vi "Extract F0.vi"(8 "Error In":errorcluster) -> (0 "Error Out":errorcluster)   [LabVIEW 2018, in "AnalysisSupport.lvlib"]
uses:
  AnalysisSupport.lvlib
  Analysis Support/Controls/F0 Extraction Test Types.ctl
  Analysis Support/Controls/F0 Extraction States.ctl
  Analysis Support/Controls/F0 Cluster.ctl
  <vilib>/Waveform/WDTOps.llb/WDT Get Waveform Subset DBL.vi
  <vilib>/Analysis/NI_AALBase.lvlib
  CollectionSupport.lvlib
panel:
  out "Selected":dbl format="%#.2g"
  out "Test-Matched Files":path[](array[path])
  out "Min":dbl
  out "Max":dbl
  out "Median":dbl
  out "Progress Bar":u8(slide) scale=0.0..10.0
  out "F0 Array (Hz)":dbl[](array[numeric]) format="%#.2g"
  out "CoV":dbl format="%.2f%%"
  out "St.Dev":dbl format="%#.2g"
  out "Mean F0 (Hz)":dbl format="%#.2g"
  in  "Trial":dbl=1.0 min=1.0 max=15.0 step=1.0
  in  "Section Duration":dbl=0.1 min=0.1 max=1.0 step=0.1
  in  "Start Second":dbl min=0.0 max=10.0 step=0.1
  in  "Remove Button":bool
  in  "ReRun Button":bool
  in  "Save  Button":bool
  in  "Test Type Select":T1 items=["Labial SGP", "Labial PTP", "Mech Mouth", "Mech Mask"]
  in  "Trial Number":i32=1 min=1 max=15 step=1
  in  "Exit Button":bool
  in  "Open Button":bool
  in  "Examine Button":bool
  in  "Extract Button":bool
  out "Audio Graph":dynamicdata(graph)
  out "Total Files":i32
  out "All Files in Directory":path[](array[path])
  # "Remove an index to change stats"
  # "Save the mean, standard deviation, & coefficient of variation to a txt file."
  # "Re-run extraction using a different section of signal"
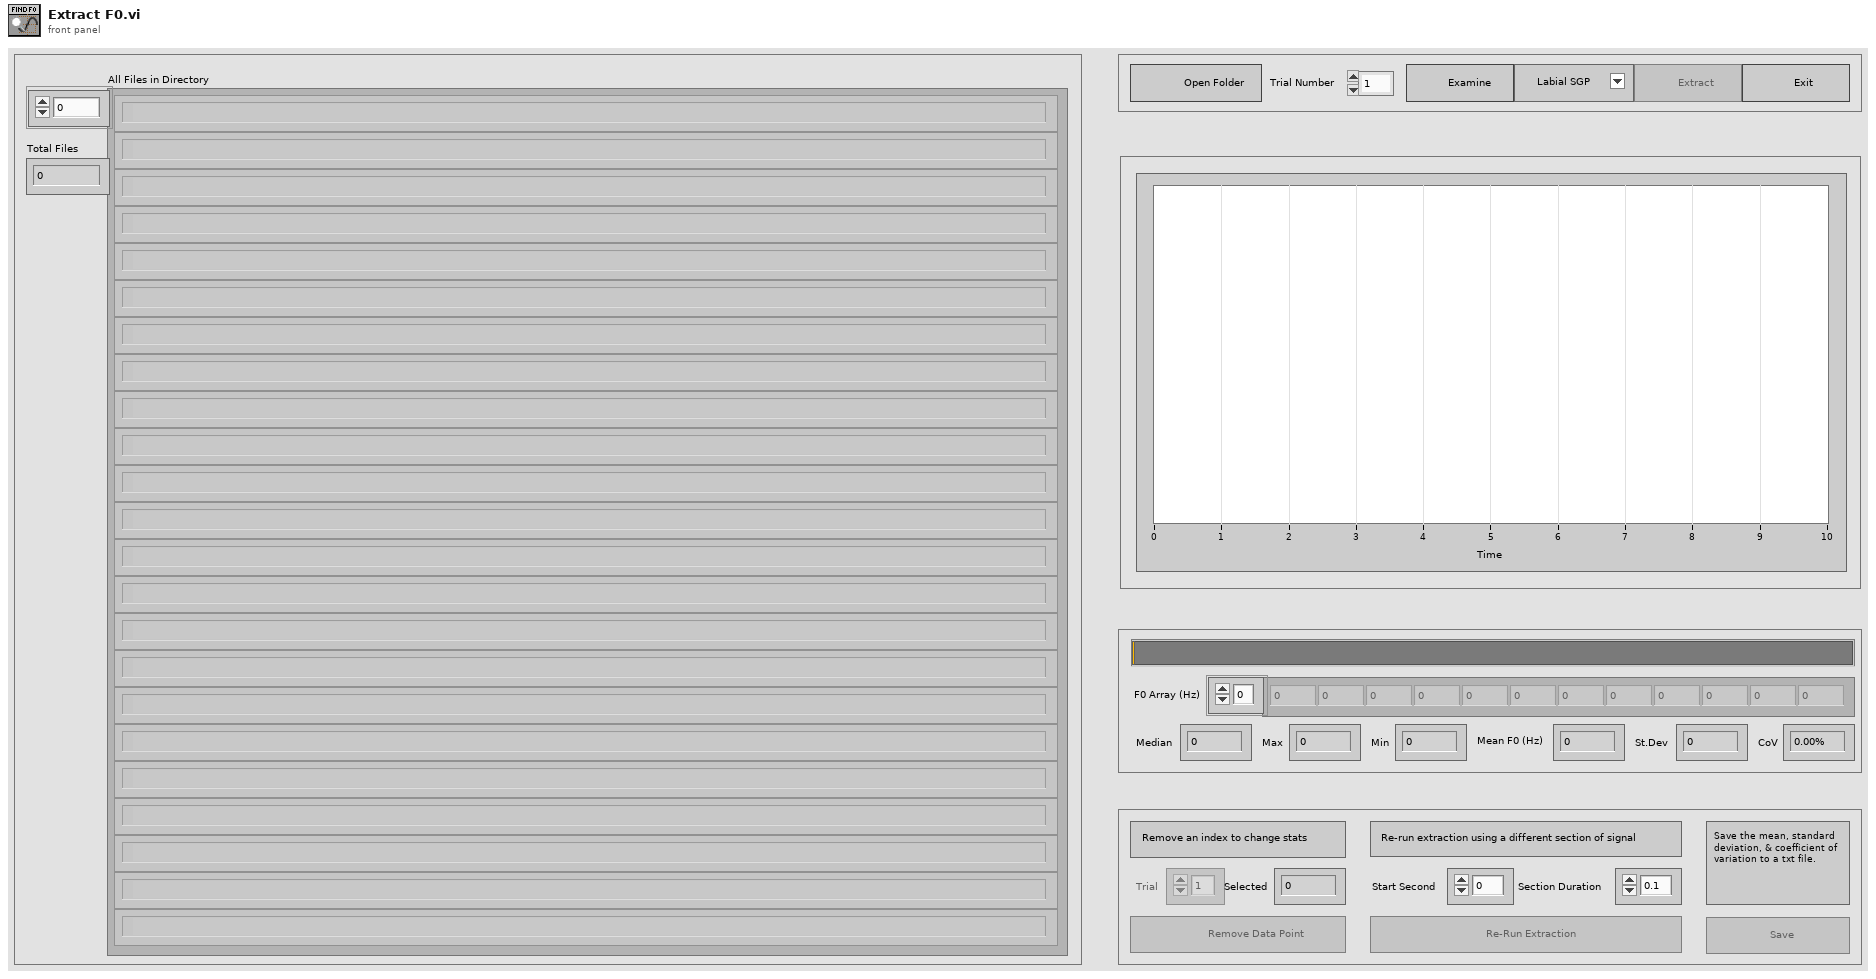
[diagram p1: front panel]
types:
  T1 = typedef "AnalysisSupport.lvlib/F0 Extraction Test Types.ctl" = u16
  T2 = typedef "AnalysisSupport.lvlib/F0 Cluster.ctl" = cluster{"F0 and Trial #":cluster{"F0 Array":dbl[], "Matched Trial #":string[]}, "Mean":dbl, "STD":dbl, "CoV":dbl, "Median":dbl, "Max":dbl, "Min":dbl, "Start Second":dbl, "Section Duration":dbl, "Total Files":i32, "Trial Number":i32, "Progress Bar Max":u8, "Selected F0":dbl, "Trial Index":dbl, "Test Type":string, "File Array":path[], "File Subset":path[], "Audio Data":dynamicdata, "References":cluster{"Trial":refnum<vi>, "Open Button":refnum<vi>, "Examine Button":refnum<vi>, "Test Type Select":refnum<vi>, "Extract Button":refnum<vi>, "Exit Button":refnum<vi>, "Remove Button":refnum<vi>, "ReRun Button":refnum<vi>, "Save  Button":refnum<vi>, "Progress Bar":refnum<vi>}}
  T3 = typedef "AnalysisSupport.lvlib/F0 Extraction States.ctl" = enum16{"Initialize", "Update", "Wait", "Open Folder", "Examine", "Extract", "Re Run", "Remove", "Save", "Exit"}
  T4 = enum8{"Enabled", "Disabled", "Disabled and Grayed Out"}
  T5 = enum16{"open", "replace", "create", "open or create", "replace or create", "replace or create with confirmation"}
  T6 = cluster{"Trial":refnum<vi>, "Open Button":refnum<vi>, "Examine Button":refnum<vi>, "Test Type Select":refnum<vi>, "Extract Button":refnum<vi>, "Exit Button":refnum<vi>, "Remove Button":refnum<vi>, "ReRun Button":refnum<vi>, "Save  Button":refnum<vi>, "Progress Bar":refnum<vi>}
  T7 = cluster{"F0 Array":dbl[], "Matched Trial #":string[]}
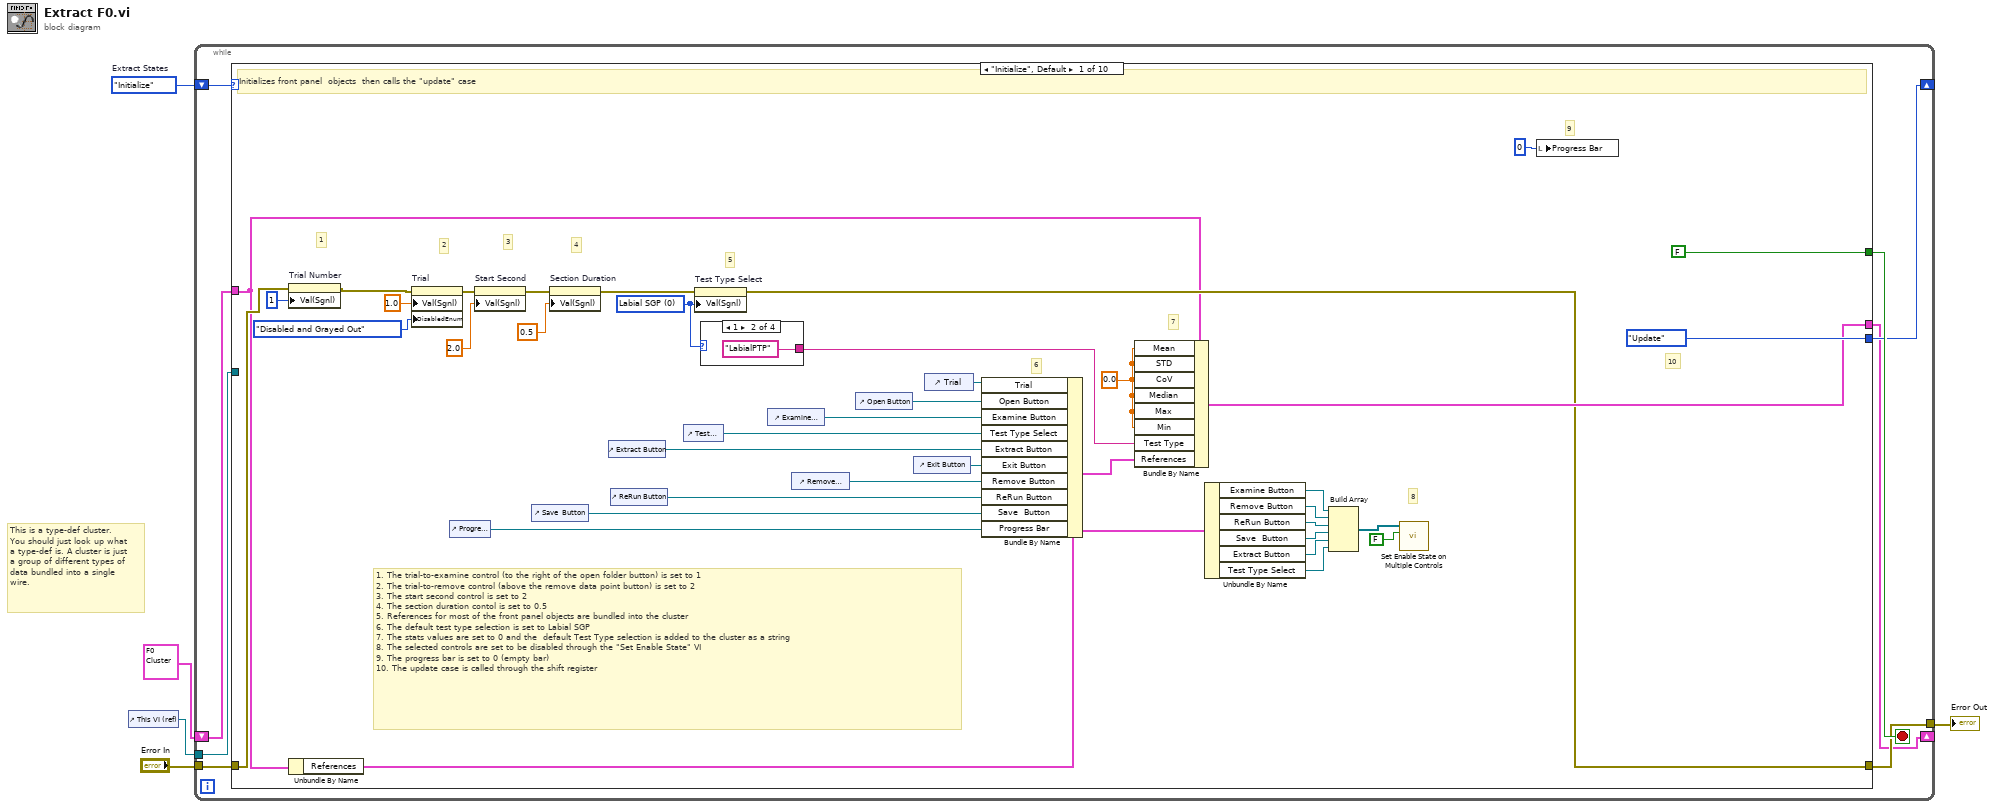
[diagram p0: block diagram]
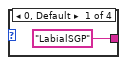
[diagram p2: hidden frame]
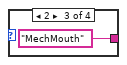
[diagram p3: hidden frame]
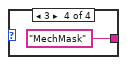
[diagram p4: hidden frame]
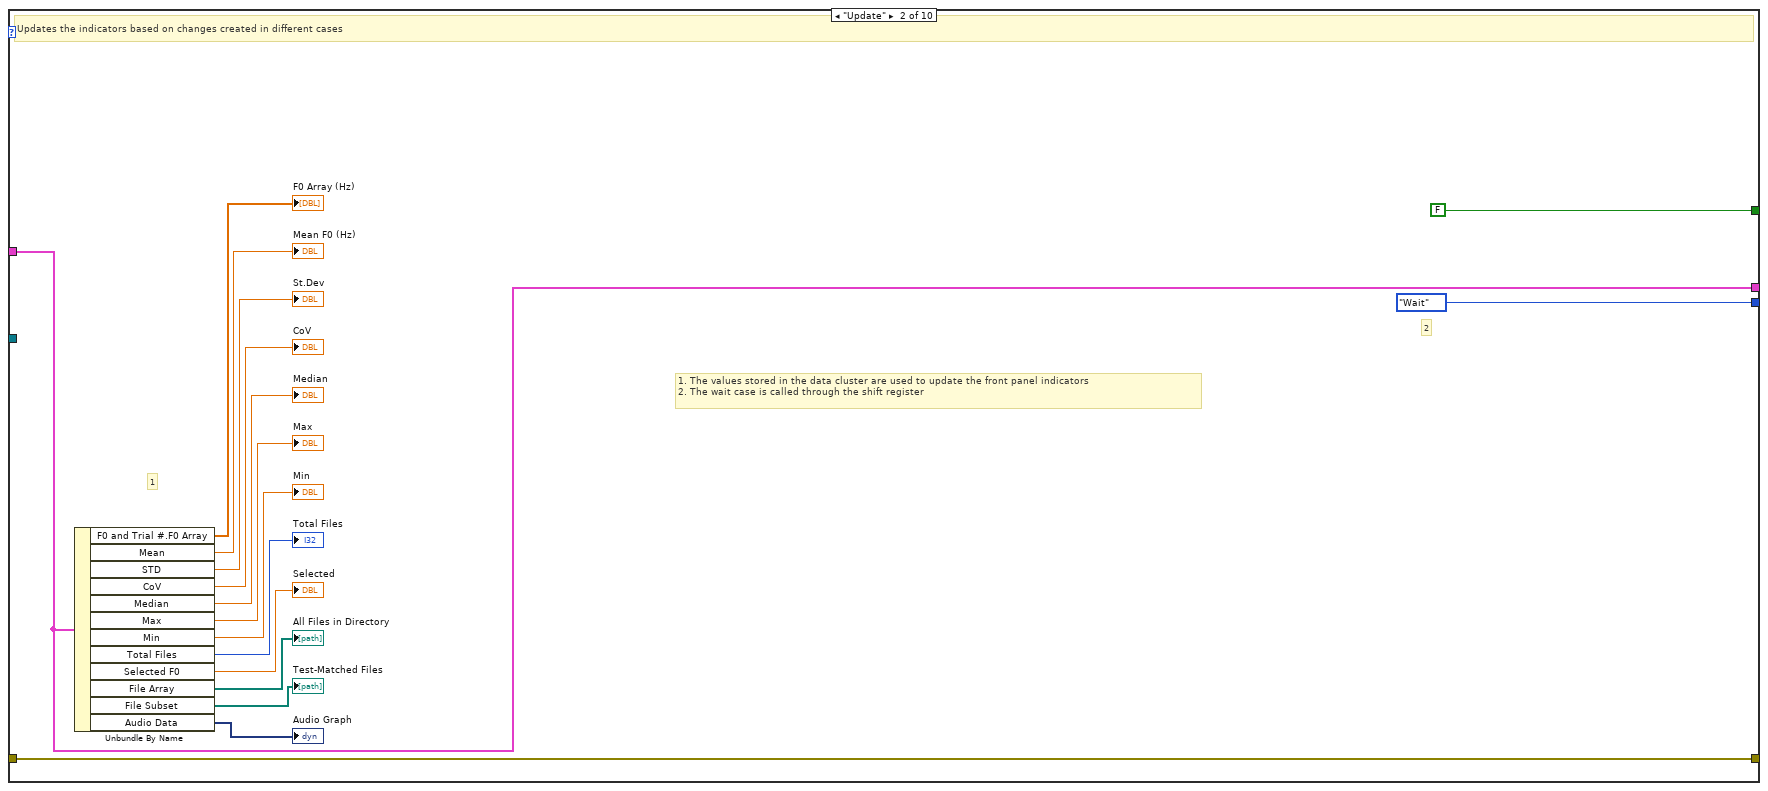
[diagram p5: hidden frame]
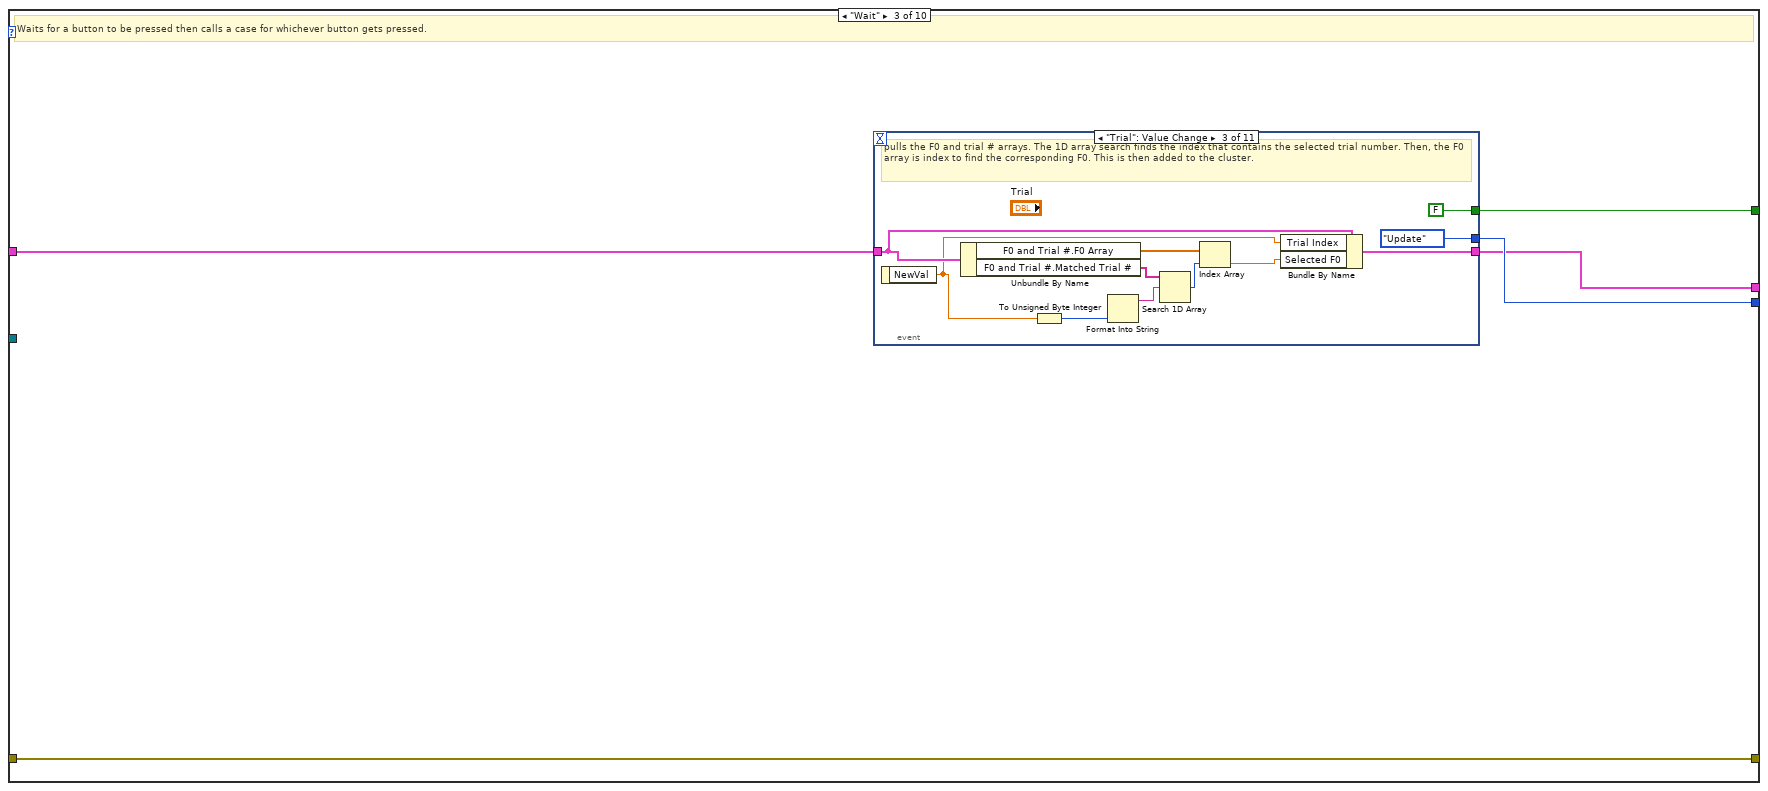
[diagram p6: hidden frame]
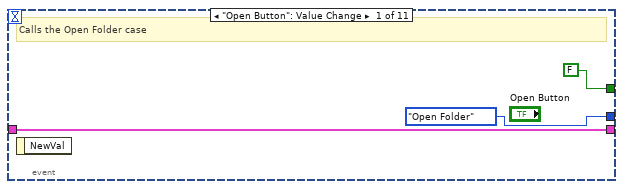
[diagram p7: hidden frame]
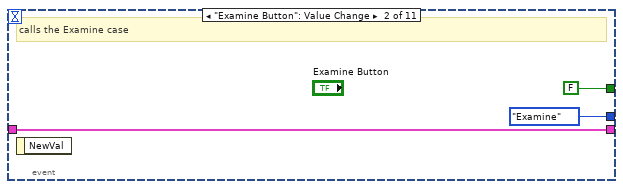
[diagram p8: hidden frame]
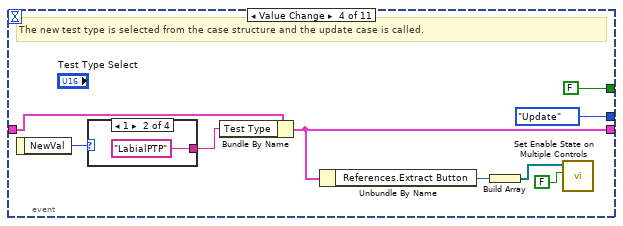
[diagram p9: hidden frame]
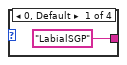
[diagram p10: hidden frame]
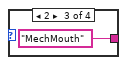
[diagram p11: hidden frame]
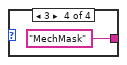
[diagram p12: hidden frame]
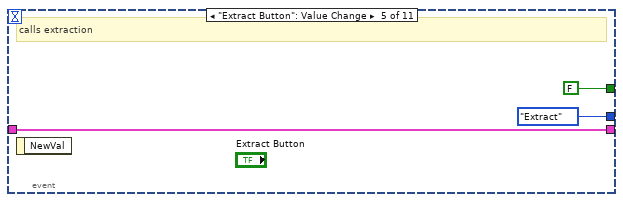
[diagram p13: hidden frame]
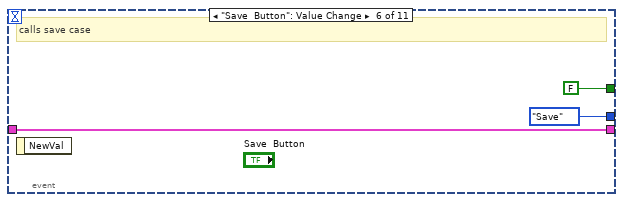
[diagram p14: hidden frame]
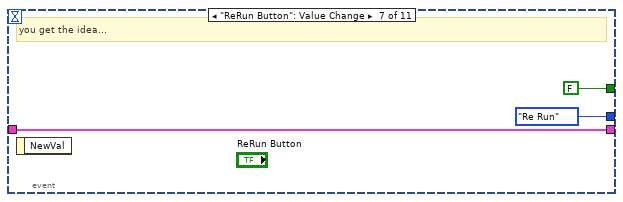
[diagram p15: hidden frame]
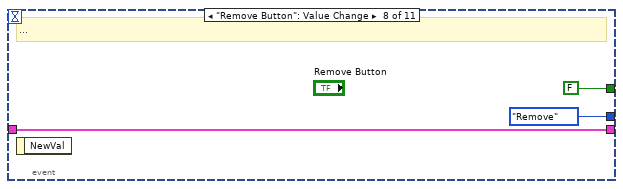
[diagram p16: hidden frame]
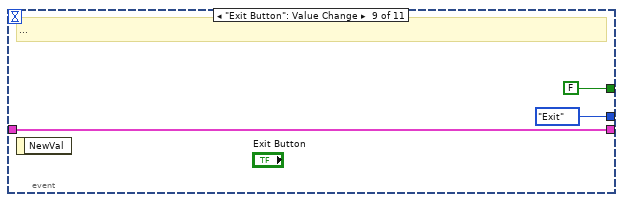
[diagram p17: hidden frame]
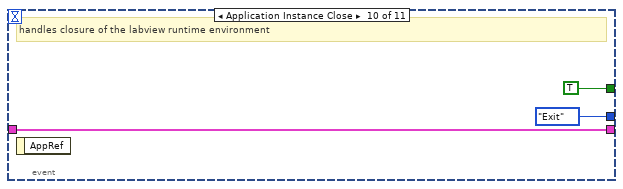
[diagram p18: hidden frame]
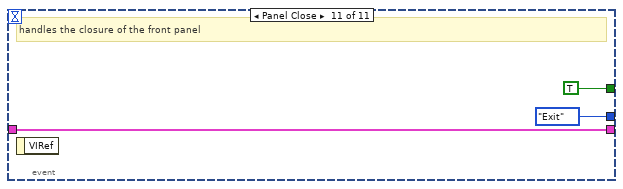
[diagram p19: hidden frame]
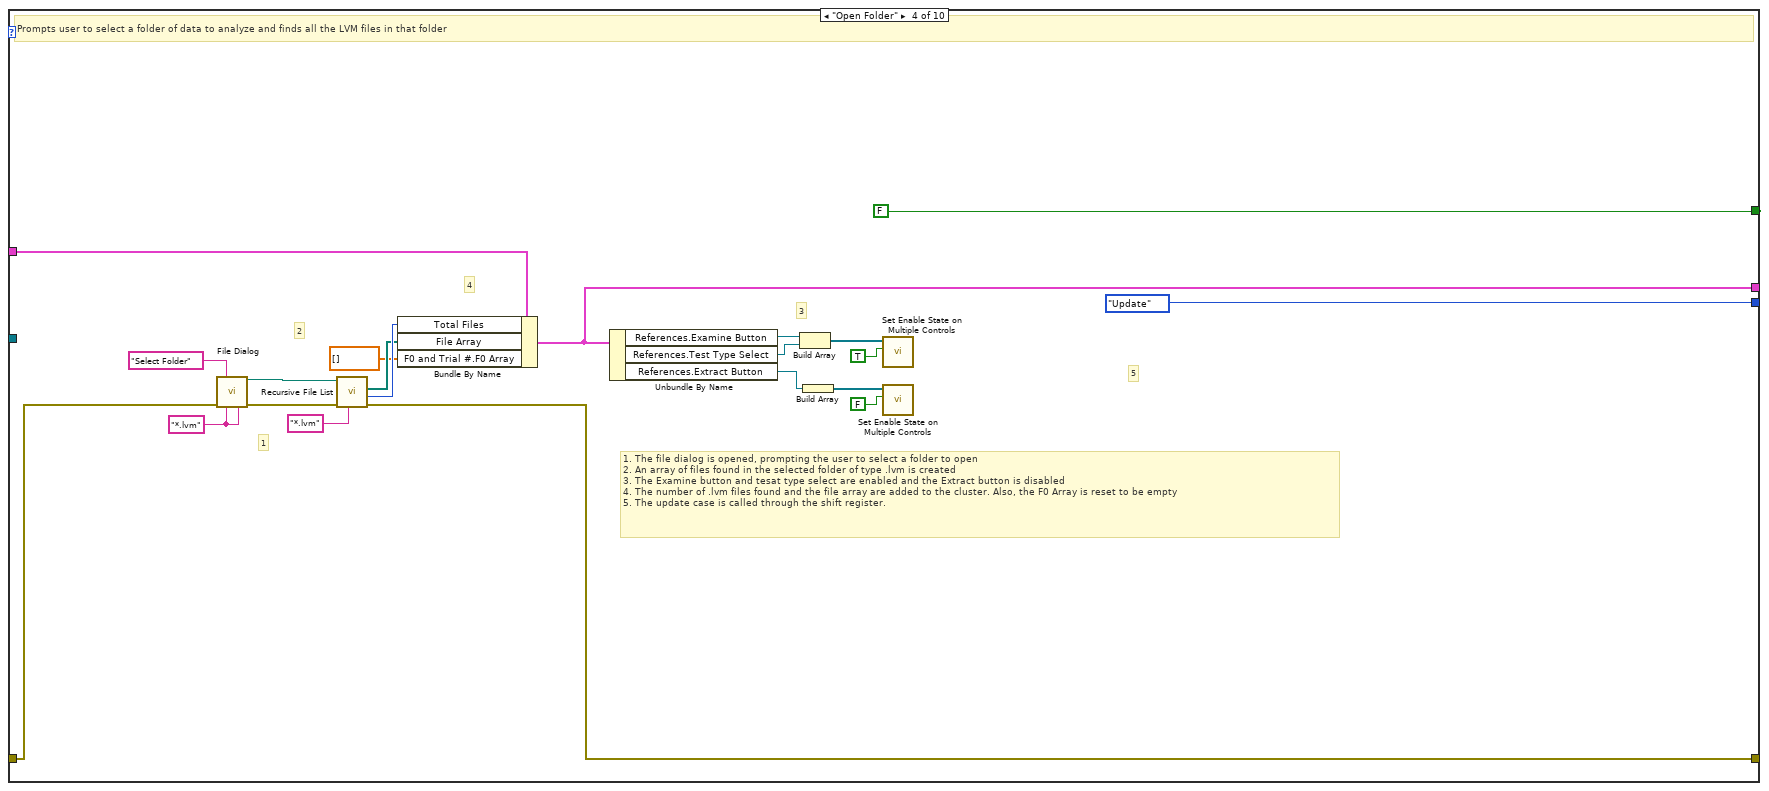
[diagram p20: hidden frame]
diagram:
  w5 = F0_Extraction_States."Initialize"  # Extract States
  # "This is a type-def cluster. You should just look up what a type-def is. A cluster is just a group of different types of data bundled into a single wire."
  n1 = control-ref of="This VI (ref)"() -> (w3:refnum<vi>)
  n2 = while {
    shift-right: [w11] -> _
    shift-left: w5 -> [w12]
    tunnel: "Error In" -> [w10]
    tunnel: w3 -> [w9]
    tunnel: [w8] -> w2
    shift-right: [w6] -> _
    shift-left: T2 {"F0 and Trial #"={"F0 Array"=[], "Matched Trial #"=[]}, "Mean"=0.0, "STD"=0.0, "CoV"=0.0, "Median"=0.0, "Max"=0.0, "Min"=0.0, "Start Second"=2.0, "Section Duration"=0.5, "Total Files"=0, "Trial Number"=0, "Progress Bar Max"=0, "Selected F0"=0.0, "Trial Index"=0.0, "Test Type"="", "File Array"=[], "File Subset"=[], "Audio Data"=[], "References"={"Trial"=refnum, "Open Button"=refnum, "Examine Button"=refnum, "Test Type Select"=refnum, "Extract Button"=refnum, "Exit Button"=refnum, "Remove Button"=refnum, "ReRun Button"=refnum, "Save  Button"=refnum, "Progress Bar"=refnum}} -> [w7]
    stop <- w13 stop-if-true
    n3 = case shown="\"Initialize\", Default" w12 {
      tunnel: [FALSE FALSE w77 FALSE FALSE FALSE FALSE FALSE FALSE TRUE] -> w13
      tunnel: [F0_Extraction_States."Update" F0_Extraction_States."Wait" w76 F0_Extraction_States."Update" F0_Extraction_States."Update" F0_Extraction_States."Update" F0_Extraction_States."Extract" F0_Extraction_States."Update" F0_Extraction_States."Wait" F0_Extraction_States."Exit"] -> w11
      tunnel: w10 -> [w36 w59 w75 w146 w150 w253 w295 w355 w403 w406]
      tunnel: w9 -> [_ _ _ _ w165 w255 _ _ _ _]
      tunnel: [w38 w59 w75 w136 w154 w221 w295 w355 w386 w406] -> w8
      tunnel: w7 -> [w35 w57 w74 w141 w159 w249 w298 w351 w364 w405]
      tunnel: [w47 w57 w73 w137 w158 w238 w297 w343 w364 w405] -> w6
      frame "Initialize", Default {
        w40 = T1 0 items=["Labial SGP", "Labial PTP", "Mech Mouth", "Mech Mask"] ("Value (Signaling)")
        w48 = 0.0 ("Mean")
        # "10"
        # "1. The trial-to-examine control (to the right of the open folder button) is set to 1\n2. The trial-to-remove control (above the remove data point button) is set to 2\n3. The start second control is set to 2\n4. The section duration contol is set to 0.5\n5. References for most of the front panel objects are bundled into the cluster\n6. The default test type selection is set to Labial SGP\n7. The stats values are set to 0 and the  default Test Type selection is added to the cluster as a string\n8. The selected controls are set to be disabled through the \"Set Enable State\" VI \n9. The progress bar is set to 0 (empty bar)\n10. The update case is called through the shift register"
        # "9"
        # "8"
        # "7"
        # "6"
        # "5"
        # "4"
        # "3"
        # "2"
        # "1"
        # "Initializes front panel  objects  then calls the \"update\" case"
        n4 = property on="Trial Number" class="DigNum (strict)"(error in=w36, "Val(Sgnl)"=1 ("Value (Signaling)")) -> (error out=w37:errorcluster)  [unwired: 1 in, 1 out]
        n5 = Unbundle By Name(w35) -> ("References"=w34:T6)
        n6 = property on="Trial" class="DigNum (strict)"(error in=w37, "Val(Sgnl)"=1.0 ("Value (Signaling)"), "DisabledEnum"=T4."Disabled and Grayed Out" ("Disabled")) -> (error out=w44:errorcluster)  [unwired: 1 in, 1 out]
        n7 = control-ref of="Progress Bar"() -> (w30:refnum<vi>)
        n8 = property on="Start Second" class="DigNum (strict)"(error in=w44, "Val(Sgnl)"=2.0 ("Start Second")) -> (error out=w43:errorcluster)  [unwired: 1 in, 1 out]
        n9 = control-ref of="Save  Button"() -> (w23:refnum<vi>)
        n10 = property on="Section Duration" class="DigNum (strict)"(error in=w43, "Val(Sgnl)"=0.5 ("Section Duration")) -> (error out=w15:errorcluster)  [unwired: 1 in, 1 out]
        n11 = control-ref of="Extract Button"() -> (w27:refnum<vi>)
        n12 = control-ref of="ReRun Button"() -> (w24:refnum<vi>)
        n13 = control-ref of="Test Type Select"() -> (w28:refnum<vi>)
        n14 = property on="Test Type Select" class="Ring (strict)"(error in=w15, "Val(Sgnl)"=w40) -> (error out=w38:errorcluster)  [unwired: 1 in, 1 out]
        n15 = case shown="1" w40 {
          tunnel: ["LabialSGP" ("regular expression") "LabialPTP" ("regular expression") "MechMouth" ("regular expression") "MechMask" ("regular expression")] -> w39
          frame 0, Default {
          }
          frame 1 {
          }
          frame 2 {
          }
          frame 3 {
          }
        }
        n16 = control-ref of="Examine Button"() -> (w31:refnum<vi>)
        n17 = control-ref of="Remove Button"() -> (w25:refnum<vi>)
        n18 = control-ref of="Open Button"() -> (w32:refnum<vi>)
        n19 = control-ref of="Exit Button"() -> (w26:refnum<vi>)
        n20 = control-ref of="Trial"() -> (w33:refnum<vi>)
        n21 = Bundle By Name(cluster=w34, "Trial"=w33, "Open Button"=w32, "Examine Button"=w31, "Test Type Select"=w28, "Extract Button"=w27, "Exit Button"=w26, "Remove Button"=w25, "ReRun Button"=w24, "Save  Button"=w23, "Progress Bar"=w30) -> (w21:T6)
        n22 = Bundle By Name(cluster=w35, "Mean"=w48, "STD"=w48, "CoV"=w48, "Median"=w48, "Max"=w48, "Min"=w48, "Test Type"=w39, "References"=w21) -> (w47:T2)
        n23 = Unbundle By Name(w21) -> ("Examine Button"=w20:refnum<vi>, "Remove Button"=w19:refnum<vi>, "ReRun Button"=w18:refnum<vi>, "Save  Button"=w17:refnum<vi>, "Extract Button"=w16:refnum<vi>, "Test Type Select"=w14:refnum<vi>)
        n24 = Build Array(w20, w19, w18, w17, w16, w14) -> (w22:refnum<vi>[])
        n25 = call "Set Enable State on Multiple Controls.vi"("Enable?"=FALSE, "Controls"=w22) -> ()  [unwired: 10 in]
        n26 = local write "Progress Bar"(u8 0 ("Progress Bar")) -> ()
      }
      frame "Update" {
        # "1. The values stored in the data cluster are used to update the front panel indicators\n2. The wait case is called through the shift register"
        # "2"
        # "1"
        # "Updates the indicators based on changes created in different cases"
        n27 = Unbundle By Name(w57) -> ("F0 and Trial #.F0 Array"=→"F0 Array (Hz)":dbl[], "Mean"=→"Mean F0 (Hz)":dbl, "STD"=→"St.Dev":dbl, "CoV"=→"CoV":dbl, "Median"=→"Median":dbl, "Max"=→"Max":dbl, "Min"=→"Min":dbl, "Total Files"=→"Total Files":i32, "Selected F0"=→"Selected":dbl, "File Array"=→"All Files in Directory":path[], "File Subset"=→"Test-Matched Files":path[], "Audio Data"=→"Audio Graph":dynamicdata)
      }
      frame "Wait" {
        # "Waits for a button to be pressed then calls a case for whichever button gets pressed."
        n28 = event shown="[2] \"Trial\": Value Change" {
          selector: _ -> [_ _ _ _ _ _ _ _ _ _ _]
          dyn-events: _ -> [_ _ _ _ _ _ _ _ _ _ _]
          timeout: _ -> [_ _ _ _ _ _ _ _ _ _ _]
          tunnel: [FALSE FALSE FALSE FALSE FALSE FALSE FALSE FALSE FALSE TRUE TRUE] -> w77
          tunnel: [F0_Extraction_States."Open Folder" F0_Extraction_States."Examine" F0_Extraction_States."Update" F0_Extraction_States."Update" F0_Extraction_States."Extract" F0_Extraction_States."Save" F0_Extraction_States."Re Run" F0_Extraction_States."Remove" F0_Extraction_States."Exit" F0_Extraction_States."Exit" F0_Extraction_States."Exit"] -> w76
          tunnel: w74 -> [w78 w81 w91 w103 w108 w111 w114 w117 w120 w123 w126]
          tunnel: [w78 w81 w90 w98 w108 w111 w114 w117 w120 w123 w126] -> w73
          event "Open Button": Value Change {
            # "Calls the Open Folder case"
            n29 = event-data() -> ()  [unwired: 1 in, 1 out]
          }
          event "Examine Button": Value Change {
            # "calls the Examine case"
            n30 = event-data() -> ()  [unwired: 1 in, 1 out]
          }
          event "Trial": Value Change {
            # "pulls the F0 and trial # arrays. The 1D array search finds the index that contains the selected trial number. Then, the F0 array is index to find the corresponding F0. This is then added to the cluster."
            n31 = event-data() -> ("NewVal"=w85:dbl)  [unwired: 1 in]
            n32 = Unbundle By Name(w91) -> ("F0 and Trial #.F0 Array"=w92:dbl[], "F0 and Trial #.Matched Trial #"=w89:string[])
            n33 = To Unsigned Byte Integer(number=w85) -> (unsigned 8bit integer=w84:u8)
            n34 = Format Into String(w84) -> (resulting string=w88:string)  [unwired: 3 in, 1 out]
            n35 = Search 1D Array(1D array=w89, element=w88) -> (index of element=w87:i32)  [unwired: 1 in]
            n36 = Index Array(array=w92, index=w87) -> (element=w86:dbl)
            n37 = Bundle By Name(cluster=w91, "Trial Index"=w85, "Selected F0"=w86) -> (w90:T2)
          }
          event Value Change {
            # "The new test type is selected from the case structure and the update case is called."
            n38 = event-data() -> ("NewVal"=w101:T1)  [unwired: 1 in]
            n39 = case shown="1" w101 {
              tunnel: ["LabialSGP" ("regular expression") "LabialPTP" ("regular expression") "MechMouth" ("regular expression") "MechMask" ("regular expression")] -> w102
              frame 0, Default {
              }
              frame 1 {
              }
              frame 2 {
              }
              frame 3 {
              }
            }
            n40 = Bundle By Name(cluster=w103, "Test Type"=w102) -> (w98:T2)
            n41 = Unbundle By Name(w98) -> ("References.Extract Button"=w97:refnum<vi>)
            n42 = Build Array(w97) -> (w96:refnum<vi>[])
            n43 = call "Set Enable State on Multiple Controls.vi"("Enable?"=FALSE, "Controls"=w96) -> ()  [unwired: 10 in]
          }
          event "Extract Button": Value Change {
            # "calls extraction"
            n44 = event-data() -> ()  [unwired: 1 in, 1 out]
          }
          event "Save  Button": Value Change {
            # "calls save case"
            n45 = event-data() -> ()  [unwired: 1 in, 1 out]
          }
          event "ReRun Button": Value Change {
            # "you get the idea..."
            n46 = event-data() -> ()  [unwired: 1 in, 1 out]
          }
          event "Remove Button": Value Change {
            # "..."
            n47 = event-data() -> ()  [unwired: 1 in, 1 out]
          }
          event "Exit Button": Value Change {
            # "..."
            n48 = event-data() -> ()  [unwired: 1 in, 1 out]
          }
          event Application Instance Close {
            # "handles closure of the labview runtime environment"
            n49 = event-data() -> ()  [unwired: 1 in, 1 out]
          }
          event Panel Close {
            # "handles the closure of the front panel"
            n50 = event-data() -> ()  [unwired: 1 in, 1 out]
          }
        }
      }
      frame "Open Folder" {
        w148 = "*.lvm" ("pattern label")
        # "3"
        # "1. The file dialog is opened, prompting the user to select a folder to open\n2. An array of files found in the selected folder of type .lvm is created\n3. The Examine button and tesat type select are enabled and the Extract button is disabled\n4. The number of .lvm files found and the file array are added to the cluster. Also, the F0 Array is reset to be empty\n5. The update case is called through the shift register."
        # "5"
        # "4"
        # "2"
        # "1"
        # "Prompts user to select a folder of data to analyze and finds all the LVM files in that folder"
        n51 = call "File Dialog"("prompt"="Select Folder", "error in"=w146, "pattern (all files)"=w148, "pattern label"=w148) -> ("selected path"=w144:path, "error out"=w145:errorcluster)  [unwired: 8 in, 2 out]
        n52 = call <vilib>:"Recursive File List.vi"("pattern"="*.lvm", "error in (no error)"=w145, "Folder Path"=w144) -> ("error out"=w136:errorcluster, "Number of Files"=w140:i32, "All Files in Dir"=w139:path[])  [unwired: 4 in, 2 out]
        n53 = Bundle By Name(cluster=w141, "Total Files"=w140, "File Array"=w139, "F0 and Trial #.F0 Array"=dbl[] [] ("F0 Array (Hz)")) -> (w137:T2)
        n54 = Unbundle By Name(w137) -> ("References.Examine Button"=w132:refnum<vi>, "References.Test Type Select"=w133:refnum<vi>, "References.Extract Button"=w130:refnum<vi>)
        n55 = Build Array(w132, w133) -> (w131:refnum<vi>[])
        n56 = Build Array(w130) -> (w129:refnum<vi>[])
        n57 = call "Set Enable State on Multiple Controls.vi"("Enable?"=TRUE, "Controls"=w131) -> ()  [unwired: 10 in]
        n58 = call "Set Enable State on Multiple Controls.vi"("Enable?"=FALSE, "Controls"=w129) -> ()  [unwired: 10 in]
      }
      frame "Examine" {
        # "1. The test type string and the full file array are unbundled from the cluster\n2. The for loop iterates through the file names searching for ones that contain the string matching the selected test type. When a match is found, it, along with the trial number, are added to arrays.\n3. If a matching file was added to the file array (the array is not empty), then the index of the selected trial-to-be-examined is found in the trial number array. This index will match the index of the file array. The file array is indexed and passed into the singal split SubVI. From there, the audio data, along with the file subset, the size of the file subset (the progress bar max), and the file number array are  bundled into the cluser. Also, the extract button is enabled.\n4. The update case is called through the shift register"
        # "4."
        # "3."
        # "2."
        # "1."
        # "finds all files of the matching test type then opens up the selected trial and extracts the audio data"
        n59 = Unbundle By Name(w159) -> ("Test Type"=w162:string, "File Array"=w161:path[])
        n60 = for {
          shift-right: [w211] -> w157
          shift-left: path[] [] ("All Files in Dir") -> [w212]
          tunnel: w162 -> [w207]
          tunnel: w161 -> [w206] mode=indexing
          shift-right: [w199] -> w152
          shift-left: string[] [] -> [w200]
          tunnel: [w198] -> w151
          tunnel: w150 -> [w198]
          # "Searches directory for files that match the test type"
          n61 = Strip Path(path=w206) -> (name=w210:string)  [unwired: 1 out]
          n62 = Match Pattern(string=w210, regular expression=w207) -> (after substring=w202:string, offset past match=w209:i32)  [unwired: 1 in, 2 out]
          n63 = Greater Than 0?(x=w209) -> (x > 0?=w208:bool)
          n64 = Match Pattern(string=w202, regular expression="Trial_") -> (after substring=w205:string)  [unwired: 1 in, 3 out]
          n65 = Match Pattern(string=w205, regular expression=".lvm") -> (before substring=w201:string)  [unwired: 1 in, 3 out]
          n66 = case shown="True" w208 {
            tunnel: w212 -> [w214 w220]
            tunnel: [w214 w219] -> w211
            tunnel: w206 -> [_ w218]
            tunnel: w201 -> [_ w217]
            tunnel: w200 -> [w213 w216]
            tunnel: [w213 w215] -> w199
            frame False {
            }
            frame True {
              n67 = Insert Into Array(array=w216, new element=w217) -> (w215:string[])  [unwired: 1 in]
              n68 = Insert Into Array(array=w220, new element=w218) -> (w219:path[])  [unwired: 1 in]
            }
          }
        }
        n69 = Empty Array?(array=w157) -> (empty?=w156:bool)
        n70 = case shown="False" w156 {
          tunnel: w165 -> [w179 _]
          tunnel: w151 -> [w171 w195]
          tunnel: "Trial Number" -> [w170 _]
          tunnel: w159 -> [w177 w197]
          tunnel: [w176 w197] -> w158
          tunnel: w157 -> [w172 _]
          tunnel: [w173 w195] -> w154
          tunnel: w152 -> [w168 _]
          frame False {
            n71 = Array Size(array=w172) -> (size(s)=w174:i32)
            n72 = Format Into String(w170) -> (resulting string=w169:string)  [unwired: 3 in, 1 out]
            n73 = To Unsigned Byte Integer(number=w174) -> (unsigned 8bit integer=w175:u8)
            n74 = Search 1D Array(1D array=w168, element=w169) -> (index of element=w166:i32)  [unwired: 1 in]
            n75 = Index Array(array=w172, index=w166) -> (element=w178:path)
            n76 = Less Than 0?(x=w166) -> (x < 0?=w167:bool)
            n77 = case shown="False" w167 {
              tunnel: w179 -> [w191 _]
              tunnel: w178 -> [w190 _]
              tunnel: w177 -> [w189 w194]
              tunnel: [w187 w194] -> w176
              tunnel: w175 -> [w186 _]
              tunnel: [w183 w193] -> w173
              tunnel: w172 -> [w182 _]
              tunnel: w171 -> [w181 w193]
              tunnel: w168 -> [w180 _]
              frame False {
                n78 = call "SplitSignals.vi"("VI reference"=w191, "Filename"=w190, "Error In"=w181) -> ("Audio"=w188:dynamicdata, "Error Out"=w185:errorcluster)  [unwired: 5 in, 6 out]
                n79 = Bundle By Name(cluster=w189, "File Subset"=w182, "Audio Data"=w188, "Progress Bar Max"=w186, "F0 and Trial #.Matched Trial #"=w180) -> (w187:T2)
                n80 = property on="Extract Button" class="Bool"(error in=w185, "DisabledEnum"=T4."Enabled" ("Disabled")) -> (error out=w183:errorcluster)  [unwired: 1 in, 1 out]
              }
              frame True {
                # "If the search 1d array function does not find the trial number, it will return a -1, thus making the Less than 0? check return a true."
                n81 = One Button Dialog(message="That trial cannot be found") -> ()  [unwired: 1 in, 1 out]
              }
            }
          }
          frame True {
            n82 = One Button Dialog(message="No files of that test type were found.") -> ()  [unwired: 1 in, 1 out]
          }
        }
      }
      frame "Extract" {
        w252 = u8 0  # Progress Bar
        w254 = dbl[] []  # F0 Array
        # "1. The progress bar max, test type string, type-matched file subset, and the F0 & trial number cluster are unbundled form the main cluster\n2. The for loop iterates through all the file names in the file subset, double checks the test type then enters the case structure\n3. Opens the files that is being read at the current iteration, extracts the audio data and converts it to a waveform. This is passed into the Get Waveform Subset function. The section of waveform starting at the start second, with a length of the section duration, is output from this function. The waveform is then converted back into dynamic data and passed into the Tone measurement express vi. The F0 is calculated here, then added to the array of F0 values. When an F0 is added, the progress bar is incremented.\n4. The index of the first trial is found and the F0 array is indexed to set the trial-to-remove value\n5. Stats are performed on the F0 array\n6. Stats are bundled into the cluster.\n7. The update case is called through the shift register"
        # "7"
        # "6"
        # "5"
        # "4"
        # "3"
        # "2"
        # "1."
        # "Extracts frequency data of the selected trial type at the specified second (default is 2) with a specific duration (defualut is 0.5)"
        n83 = Unbundle By Name(w249) -> ("Progress Bar Max"=w237:u8, "Test Type"=w240:string, "File Subset"=w239:path[], "F0 and Trial #"=w236:T7, "References"=w231:T6)
        n84 = for {
          tunnel: w240 -> [w270]
          tunnel: [w262] -> w221
          tunnel: w255 -> [w269]
          shift-right: [w267] -> w248
          shift-left: w254 -> [w268]
          tunnel: w253 -> [w261]
          shift-right: [w260] -> _
          shift-left: w252 -> [w264]
          tunnel: w237 -> [w259]
          tunnel: w239 -> [w258] mode=indexing
          n85 = Strip Path(path=w258) -> (name=w273:string)  [unwired: 1 out]
          n86 = Match Pattern(string=w273, regular expression=w270) -> (offset past match=w272:i32)  [unwired: 1 in, 3 out]
          n87 = Greater Than 0?(x=w272) -> (x > 0?=w271:bool)
          n88 = To Double Precision Float(number=w259) -> (double precision float=w266:dbl)
          n89 = case shown="True" w271 {
            tunnel: [w275 w287] -> w263
            tunnel: w269 -> [_ w294]
            tunnel: w268 -> [w276 w286]
            tunnel: [w276 w285] -> w267
            tunnel: [w274 w282] -> w260
            tunnel: w261 -> [w275 w281]
            tunnel: w264 -> [w274 w280]
            tunnel: w258 -> [_ w277]
            frame False {
              # "Nothing happens here"
            }
            frame True {
              w290 = u16 1 items=["Samples", "Relative Time"] ("start/duration format")
              n90 = call "SplitSignals.vi"("VI reference"=w294, "Filename"=w277, "Error In"=w281) -> ("Audio"=w292:dynamicdata, "Error Out"=w288:errorcluster)  [unwired: 5 in, 6 out]
              n91 = call "Convert from Dynamic Data"("Dynamic Data Type"=w292) -> ("Waveform"=w291:waveform(dbl))  [unwired: 3 in]
              n92 = call-poly <vilib>:"Get Waveform Subset.vi"("start/duration format"=w290, "duration"="Section Duration", "start samples/time"="Start Second", "waveform in"=w291) -> ("waveform out"=w293:waveform(dbl))  [unwired: 2 in, 3 out]
              n93 = call "Convert to Dynamic Data"("Waveform"=w293) -> ("Dynamic Data Type"=w289:dynamicdata)  [unwired: 3 in]
              n94 = call "Tone Measurements"("error in (no error)"=w288, "Signals"=w289) -> ("error out"=w287:errorcluster, "Frequency"=w284:dynamicdata)  [unwired: 8 in]
              n95 = Increment(x=w280) -> (x+1=w282:u8)
              n96 = call "Convert from Dynamic Data2"("Dynamic Data Type"=w284) -> ("Scalar"=w283:dbl)  [unwired: 3 in]
              n97 = Insert Into Array(array=w286, new element=w283) -> (w285:dbl[])  [unwired: 1 in]
            }
          }
          "Progress Bar" <- w260
          n98 = property on="Progress Bar" class="Slide (strict)"(error in=w263, "Scale.Maximum"=w266, "Scale.Minimum"=0.0 ("Scale.Range:Minimum")) -> (error out=w262:errorcluster)  [unwired: 1 in, 1 out]
        }
        n99 = Unbundle By Name(w231) -> ("Trial"=w230:refnum<vi>, "Remove Button"=w229:refnum<vi>, "ReRun Button"=w228:refnum<vi>, "Save  Button"=w227:refnum<vi>, "Extract Button"=w224:refnum<vi>)
        n100 = Unbundle By Name(w236) -> ("Matched Trial #"=w235:string[])
        n101 = Build Array(w230, w229, w228, w227) -> (w225:refnum<vi>[])
        n102 = Build Array(w224) -> (w223:refnum<vi>[])
        n103 = Format Into String(1 ("index")) -> (resulting string=w233:string)  [unwired: 3 in, 1 out]
        n104 = call "Set Enable State on Multiple Controls.vi"("Enable?"=TRUE, "Controls"=w225) -> ()  [unwired: 10 in]
        n105 = call "Set Enable State on Multiple Controls.vi"("Enable?"=FALSE, "Controls"=w223) -> ()  [unwired: 10 in]
        n106 = Search 1D Array(1D array=w235, element=w233) -> (index of element=w232:i32)  [unwired: 1 in]
        n107 = call <vilib>:"Std Deviation and Variance.vi"("X"=w248) -> ("mean"=w247:dbl, "standard deviation"=w246:dbl)  [unwired: 1 in, 1 out]
        n108 = call <vilib>:"Median.vi"("X"=w248) -> ("median"=w244:dbl)  [unwired: 1 out]
        n109 = Index Array(array=w248, index=w232) -> (element=w241:dbl)
        n110 = Divide(x=w246, y=w247) -> (x/y=w251:dbl)
        n111 = Array Max & Min(array=w248) -> (max value=w243:dbl, min value=w242:dbl)  [unwired: 2 out]
        n112 = Multiply(x=w251, y=100.0) -> (x*y=w245:dbl)
        n113 = Bundle By Name(cluster=w249, "F0 and Trial #.F0 Array"=w248, "Mean"=w247, "STD"=w246, "CoV"=w245, "Median"=w244, "Max"=w243, "Min"=w242, "Selected F0"=w241) -> (w238:T2)
      }
      frame "Re Run" {
        # "3."
        # "2."
        # "1."
        # "Basically the same thing as examine except it doesn't open a trial, just reloads the file subset array then calls extraction"
        n114 = Unbundle By Name(w298) -> ("Test Type"=w305:string, "File Array"=w304:path[])  [unwired: 1 out]
        n115 = for {
          shift-right: [w327] -> w302
          shift-left: path[] [] ("All Files in Dir") -> [w328]
          tunnel: w305 -> [w323]
          tunnel: w304 -> [w322] mode=indexing
          shift-right: [w315] -> w299
          shift-left: string[] [] -> [w316]
          # "Searches directory for files that match the test type"
          n116 = Strip Path(path=w322) -> (name=w326:string)  [unwired: 1 out]
          n117 = Match Pattern(string=w326, regular expression=w323) -> (after substring=w318:string, offset past match=w325:i32)  [unwired: 1 in, 2 out]
          n118 = Greater Than 0?(x=w325) -> (x > 0?=w324:bool)
          n119 = Match Pattern(string=w318, regular expression="Trial_") -> (after substring=w321:string)  [unwired: 1 in, 3 out]
          n120 = Match Pattern(string=w321, regular expression=".lvm") -> (before substring=w317:string)  [unwired: 1 in, 3 out]
          n121 = case shown="True" w324 {
            tunnel: w328 -> [w330 w336]
            tunnel: [w330 w335] -> w327
            tunnel: w322 -> [_ w334]
            tunnel: w317 -> [_ w333]
            tunnel: w316 -> [w329 w332]
            tunnel: [w329 w331] -> w315
            frame False {
            }
            frame True {
              n122 = Insert Into Array(array=w332, new element=w333) -> (w331:string[])  [unwired: 1 in]
              n123 = Insert Into Array(array=w336, new element=w334) -> (w335:path[])  [unwired: 1 in]
            }
          }
        }
        n124 = Empty Array?(array=w302) -> (empty?=w301:bool)
        n125 = case shown="False" w301 {
          tunnel: w298 -> [w312 w314]
          tunnel: [w311 w314] -> w297
          tunnel: w302 -> [w308 _]
          tunnel: w299 -> [w307 _]
          frame False {
            n126 = Array Size(array=w308) -> (size(s)=w309:i32)
            n127 = To Unsigned Byte Integer(number=w309) -> (unsigned 8bit integer=w310:u8)
            n128 = Bundle By Name(cluster=w312, "File Subset"=w308, "Progress Bar Max"=w310, "F0 and Trial #.Matched Trial #"=w307) -> (w311:T2)
          }
          frame True {
            n129 = One Button Dialog(message="No files of that test type were found.") -> ()  [unwired: 1 in, 1 out]
          }
        }
      }
      frame "Remove" {
        # "1. The trial-to-remove number, the F0 array, and the trial # array are unbundled from the cluster\n2. The index of the selected trial number is found in the trial # array\n3. The trial is deleted from both the F0 array and the trial number array.\n4. Stats are recalculated\n5. Stats and arrays are bundled into the cluster\n6. The update case is called through the shift register"
        # "6"
        # "5"
        # "4"
        # "3"
        # "2"
        # "1"
        # "removes the selected index from the F0 array"
        n130 = Unbundle By Name(w351) -> ("Trial Index"=w337:dbl, "F0 and Trial #.F0 Array"=w352:dbl[], "F0 and Trial #.Matched Trial #"=w342:string[])
        n131 = To Unsigned Byte Integer(number=w337) -> (unsigned 8bit integer=w338:u8)
        n132 = Format Into String(w338) -> (resulting string=w341:string)  [unwired: 3 in, 1 out]
        n133 = Search 1D Array(1D array=w342, element=w341) -> (index of element=w340:i32)  [unwired: 1 in]
        n134 = Delete From Array "Delete From Array"(array=w352, index=w340) -> (array with subset deleted=w350:dbl[])  [unwired: 1 in, 1 out]
        n135 = Delete From Array "Delete From Array"(array=w342, index=w340) -> (array with subset deleted=w339:string[])  [unwired: 1 in, 1 out]
        n136 = call <vilib>:"Std Deviation and Variance.vi"("X"=w350) -> ("mean"=w349:dbl, "standard deviation"=w348:dbl)  [unwired: 1 in, 1 out]
        n137 = call <vilib>:"Median.vi"("X"=w350) -> ("median"=w346:dbl)  [unwired: 1 out]
        n138 = Divide(x=w348, y=w349) -> (x/y=w354:dbl)
        n139 = Array Max & Min(array=w350) -> (max value=w345:dbl, min value=w344:dbl)  [unwired: 2 out]
        n140 = Multiply(x=w354, y=100.0) -> (x*y=w347:dbl)
        n141 = Bundle By Name(cluster=w351, "F0 and Trial #.F0 Array"=w350, "Mean"=w349, "STD"=w348, "CoV"=w347, "Median"=w346, "Max"=w345, "Min"=w344, "F0 and Trial #.Matched Trial #"=w339) -> (w343:T2)
      }
      frame "Save" {
        w362 = "%s" ("format string")
        w360 = "\t"
        w358 = "\r\n"
        w391 = "*.txt" ("pattern label")
        # "8"
        # "1. The cluster is unbundled\n2. The f0 array and the trial # array are converted into spreadhseet strings\n3. The subject number is determined from the first file name in the array.  It is found after Subject- and before _Condition. This is then concatonated with other strings to create the default file name of Subject-#_TestType-F0 Data\n4. The file name is concatonated with the date and passed into the format into string function. \n5. The file dialog is opened to prompt the user with a save location.\n6. The data and headers are compiled into 1 string.\n7. A text file is created and the compiled string is written to it.\n8. The wait case is called through the shift register"
        # "7"
        # "6"
        # "5"
        # "3"
        # "4"
        # "2"
        # "1"
        # "Saves the mead, STD, and CoV of the F0 array to a text file"
        n142 = Unbundle By Name(w364) -> ("File Subset"=w370:path[], "F0 and Trial #.F0 Array"=w368:dbl[], "Mean"=w369:dbl, "STD"=w367:dbl, "CoV"=w366:dbl, "Test Type"=w365:string, "F0 and Trial #.Matched Trial #"=w363:string[])
        n143 = Array To Spreadsheet String(array=w363, 3:w362) -> (spreadsheet string=w361:string)  [unwired: 1 in]
        n144 = Array To Spreadsheet String(array=w368, 3:w362) -> (spreadsheet string=w377:string)  [unwired: 1 in]
        n145 = Index Array(array=w370, index=0) -> (element=w401:path)
        n146 = Strip Path(path=w401) -> (name=w400:string)  [unwired: 1 out]
        n147 = Match Pattern(string=w400, regular expression="Subject-") -> (after substring=w396:string)  [unwired: 1 in, 3 out]
        n148 = Match Pattern(string=w396, regular expression="_Condition") -> (before substring=w394:string)  [unwired: 1 in, 3 out]
        n149 = Get Date/Time In Seconds() -> (seconds since 1Jan1904=w382:timestamp)
        n150 = Get Date/Time String(seconds (now)=w382) -> (date string=w374:string)  [unwired: 2 in, 1 out]
        n151 = Concatenate Strings("Subject-" ("string"), w394, "_" ("string"), w365, "-F0 Data" ("string")) -> (w371:string)
        n152 = Concatenate Strings(w371, "\t", w374, "\r\n") -> (w372:string)
        n153 = call "File Save"("default name"=w371, "error in"=w403, "pattern (all files)"=w391, "pattern label"=w391) -> ("selected path"=w390:path, "error out"=w389:errorcluster)  [unwired: 8 in, 2 out]
        n154 = Open/Create/Replace File(file path (use dialog)=w390, error in=w389, operation (0:open)=T5."replace or create") -> (refnum out=w383:refnum<file>, error out=w388:errorcluster)  [unwired: 3 in, 1 out]
        n155 = Format Into String(initial string=w372, w358, "Trial" ("input 1"), w360, w361, "F0 Values" ("input 2"), w360, w377, "Mean" ("input 5"), w360, w369, w358, "St.Dev" ("input 8"), w360, w367, w358, "CoV (%)" ("input 5"), w360, w366) -> (resulting string=w379:string)  [unwired: 2 in, 1 out]
        n156 = Write to Text File(file (use dialog)=w383, text=w379, error in=w388) -> (refnum out=w385:refnum<file>, error out=w387:errorcluster)  [unwired: 1 in, 1 out]
        n157 = Close File(refnum=w385, error in=w387) -> (error out=w386:errorcluster)  [unwired: 1 out]
      }
      frame "Exit" {
        # "It doesn't matter what case you call here since the while loop will be stopping"
        # "Exits"
      }
    }
  }
  "Error Out" <- w2
